vi "Arm Hardware.vi"(8 "error in (no error)":errorcluster, 9 "Request type":T1=enum."User command", 11 "Red Pitaya Digitizer in":refnum<class "Red Pitaya Digitizer.lvclass">) -> (0 "error out":errorcluster, 3 "Red Pitaya Digitizer out":refnum<class "Red Pitaya Digitizer.lvclass">)   [LabVIEW 2024, in "Red Pitaya Digitizer.lvclass"]
uses:
  Red Pitaya Digitizer.lvclass
  C:/GitHub/NHMFL_Core/Libraries/Instruments/Pulse Driver/Lockin Digitizer Driver/Lockin Digitizer Driver.lvclass
  C:/GitHub/NHMFL_Core/Libraries/Instruments/Pulse Driver/Pulse Driver.lvclass
  Red Pitaya Digitizer.lvclass/Red Pitaya Digitizer.ctl
  Instruments/Pulse Driver/Pulse Driver.lvclass/Pulse Driver.ctl
  RP Core/RP Instrument/RP Instrument.lvclass/RP Instrument.ctl
  RP Core/RP Instrument/RP Instrument.lvclass
  <vilib>/Utility/miscctls.llb/LVMapReplaceAction.ctl
  LabActor/Controllers/Process Controller/Request type.ctl
panel:
  out "key not found?":bool
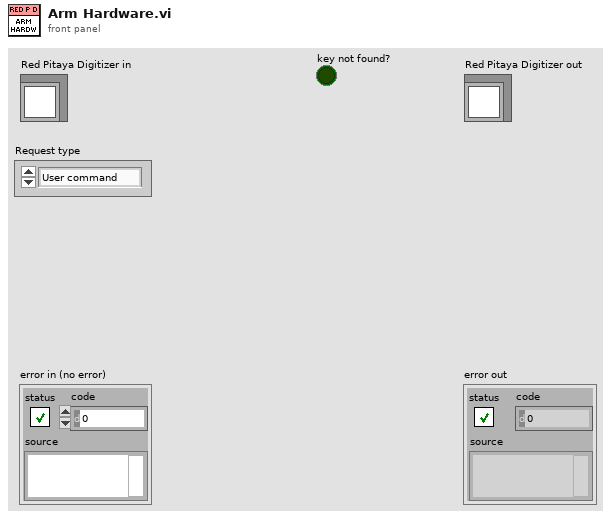
[diagram p1: front panel]
types:
  T1 = typedef "Request type.ctl" = enum16{"Process complete", "User command", "Auto-restart", "Error"}
  T2 = typedef "LVMapReplaceAction.ctl" = enum32{"Modify Entry only if found", "Add or Modify Entry", "Delete Entry"}
  T3 = typedef "Pusle Driver Configuration.ctl" = cluster{"Post-trigger delay":dbl, "Post-trigger duration":dbl, "Rate":dbl, "Ranges":dbl[], "Re-name channels":string[], "Active channels":string, "External clock":bool}
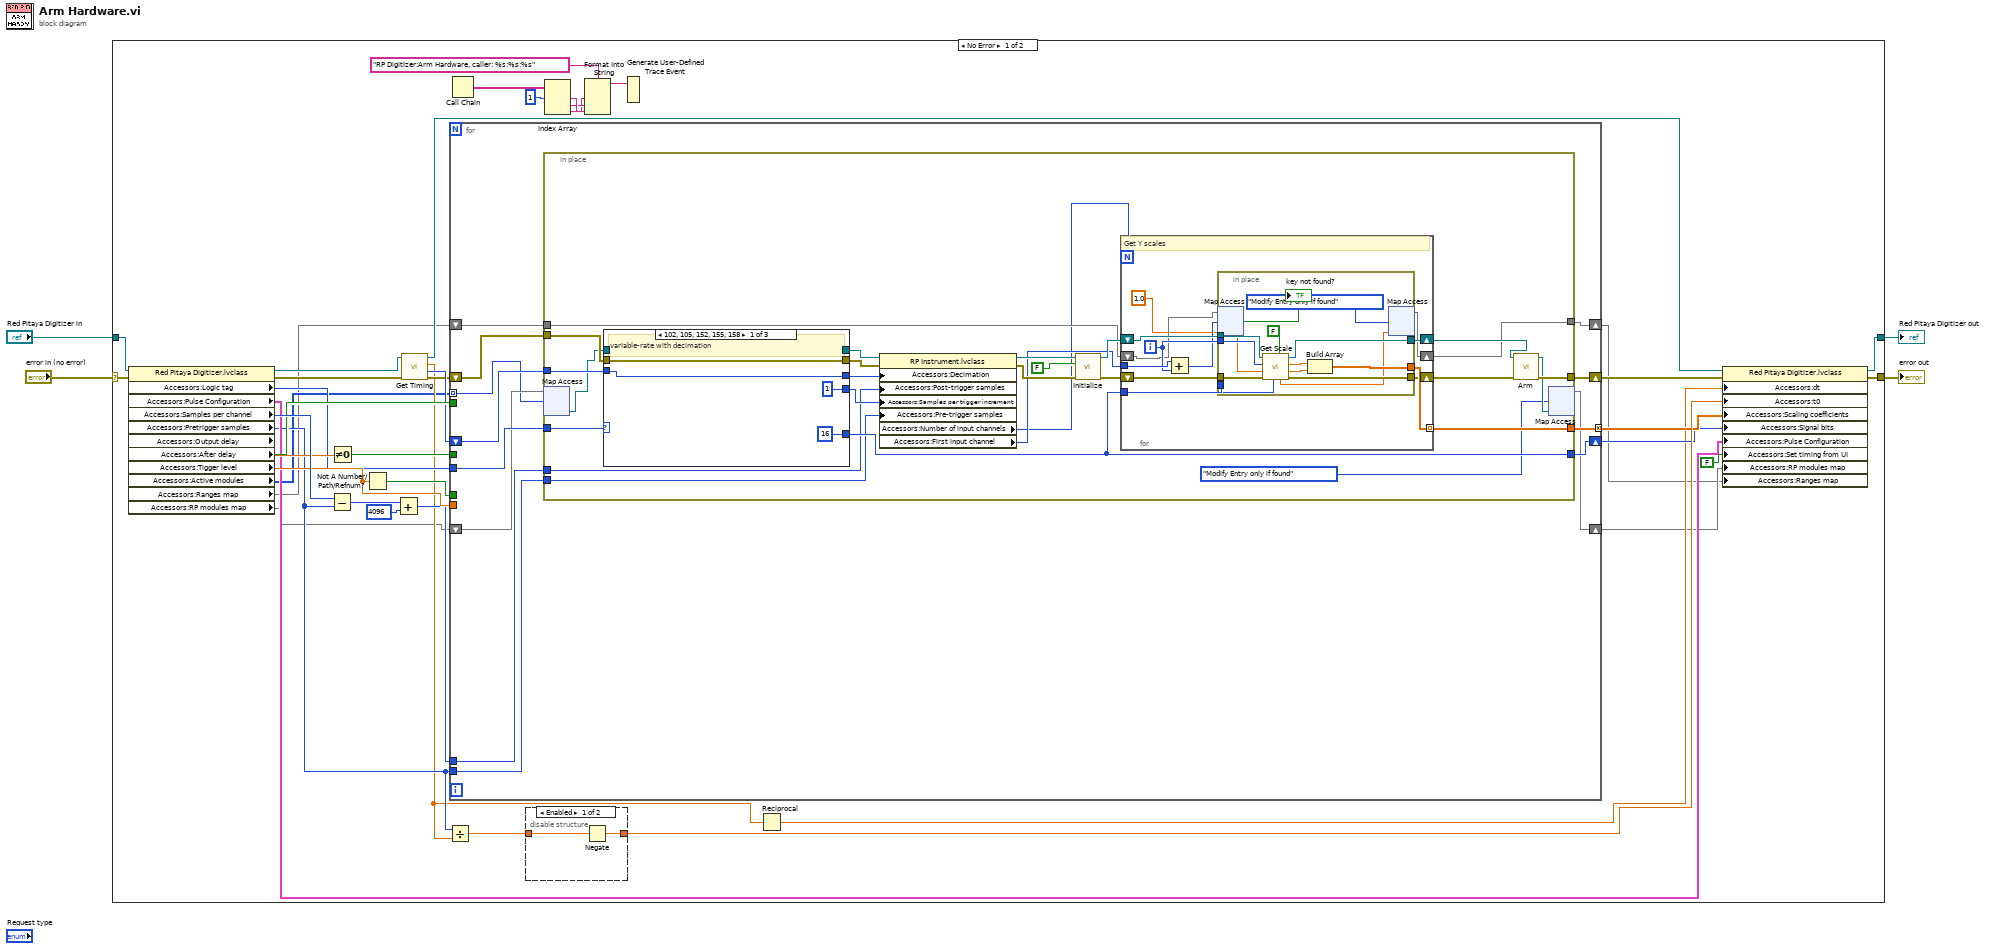
[diagram p0: block diagram]
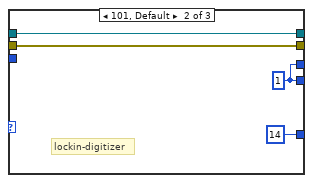
[diagram p3: hidden frame]
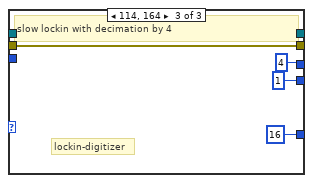
[diagram p4: hidden frame]
diagram:
  n1 = case shown="No Error" "error in (no error)" {
    selector: "error in (no error)" -> [w36 w128]
    tunnel: "Red Pitaya Digitizer in" -> [w45 w129]
    tunnel: [w41 w128] -> w2
    tunnel: [w40 w129] -> w1
    frame No Error {
      n2 = property class="Red Pitaya Digitizer.lvclass"(reference=w45, error in=w36) -> (reference out=w23:refnum<class "Red Pitaya Digitizer.lvclass">, error out=w26:errorcluster, "Accessors:Logic tag"=w28:u16, "Accessors:Pulse Configuration"=w21:T3, "Accessors:Samples per channel"=w44:i32, "Accessors:Pretrigger samples"=w11:i32, "Accessors:Output delay"=w33:dbl, "Accessors:After delay"=w32:bool, "Accessors:Tigger level"=w30:dbl, "Accessors:Active modules"=w9:i32[], "Accessors:Ranges map"=w8:map{i32, dbl}, "Accessors:RP modules map "=w7:map{i32, refnum<class "RP Instrument.lvclass">})
      n3 = Subtract(x=w44, y=w11) -> (x-y=w43:i32)
      n4 = Not Equal To 0?(x=w33) -> (x != 0?=w34:bool)
      n5 = Not A Number/Path/Refnum?(number/path/refnum=w30) -> (NaN/Path/Refnum?=w31:bool)
      n6 = Add(x=w43, y=4096) -> (x+y=w13:i32)
      n7 = call-dynamic "Get Timing.vi"("error in (no error)"=w26, "Red Pitaya Digitizer in"=w23) -> ("error out"=w24:errorcluster, "Decimation"=w25:i32, "Rate"=w10:dbl, "Red Pitaya Digitizer out"=w22:refnum<class "Red Pitaya Digitizer.lvclass">)  [unwired: 6 in]
      n8 = Divide(x=w11, y=w10) -> (x/y=w39:dbl)
      n9 = for {
        tunnel: w13 -> [w61]
        tunnel: [w59] -> w37 mode=concatenating
        tunnel: w28 -> [w57]
        tunnel: w34 -> [_]
        tunnel: w32 -> [_]
        tunnel: w31 -> [_]
        tunnel: w30 -> [_]
        shift-right: [w60] -> w42
        shift-left: w24 -> [w56]
        shift-right: [w58] -> w35
        shift-left: w25 -> [w55]
        tunnel: w11 -> [w54]
        tunnel: w9 -> [w51] mode=indexing
        shift-right: [w50] -> w6
        shift-left: w7 -> [w52]
        shift-right: [w49] -> w5
        shift-left: w8 -> [w53]
        n10 = in-place {
          in-place-border: w61 -> [w64]
          in-place-border: [w85] -> w60
          in-place-border: [w84] -> w59
          in-place-border: [w82] -> w58
          in-place-border: w57 -> [w81]
          in-place-border: w56 -> [w76]
          in-place-border: w55 -> [w73]
          in-place-border: w54 -> [w72]
          in-place-border: w53 -> [w70]
          in-place-border: [w62] -> w49
          n11 = in-place-map #1(w52, w51) -> (w67:refnum<class "RP Instrument.lvclass">)  [unwired: 1 in, 1 out]
          n12 = case shown="102, 105, 152, 155, 158" w81 {
            tunnel: [16 ("Signal bits") 14 ("Signal bits") 16 ("Signal bits")] -> w82
            tunnel: [1 ("Samples per trigger increment") w93 1 ("Samples per trigger increment")] -> w83
            tunnel: w73 -> [w88 _ _]
            tunnel: w67 -> [w90 w95 w99]
            tunnel: [w90 w95 w99] -> w75
            tunnel: w76 -> [w89 w94 w98]
            tunnel: [w89 w94 w98] -> w74
            tunnel: [w88 w93 4 ("Samples per trigger increment")] -> w63
            frame 102, 105, 152, 155, 158 {
              # "variable-rate with decimation"
            }
            frame 101, Default {
              w93 = 1 ("Samples per trigger increment")
              # "lockin-digitizer"
            }
            frame 114, 164 {
              # "lockin-digitizer"
              # "slow lockin with decimation by 4"
            }
          }
          n13 = property class="RP Instrument.lvclass"(reference=w75, error in=w74, "Accessors:Decimation"=w63, "Accessors:Post-trigger samples"=w64, "Accessors:Samples per trigger increment "=w83, "Accessors:Pre-trigger samples"=w72) -> (reference out=w87:refnum<class "RP Instrument.lvclass">, error out=w86:errorcluster, "Accessors:Number of input channels"=w68:i32, "Accessors:First input channel"=w69:i32)
          n14 = call-dynamic "Initialize.vi"("error in (no error)"=w86, "Reset"=FALSE, "RP Instrument in"=w87) -> ("error out"=w79:errorcluster, "RP Instrument out"=w80:refnum<class "RP Instrument.lvclass">)  [unwired: 7 in]
          n15 = for {
            N: w68 -> [_]
            tunnel: [w113] -> w84 mode=indexing
            tunnel: w82 -> [w110]
            shift-right: [w109] -> w77
            shift-left: w80 -> [w112]
            shift-right: [w108] -> w78
            shift-left: w79 -> [w111]
            tunnel: w69 -> [w107]
            shift-right: [w102] -> w62
            shift-left: w70 -> [w105]
            i -> [w106]
            # "Get Y scales"
            n16 = Add(x=w107, y=w106) -> (x+y=w104:i32)
            n17 = in-place {
              in-place-border: [w127] -> w113
              in-place-border: w112 -> [w126]
              in-place-border: w111 -> [w125]
              in-place-border: w110 -> [w122]
              in-place-border: [w121] -> w109
              in-place-border: [w120] -> w108
              in-place-border: w106 -> [w119]
              n18 = in-place-map #2(w105, w104, 1.0 ("default value")) -> (w117:dbl, →"key not found?":bool)
              n19 = call-dynamic "Get Scale.vi"("Read calibration"=FALSE, "Signal bits"=w122, "error in (no error)"=w125, "Range"=w117, "Channel"=w119, "RP Instrument in"=w126) -> ("error out"=w120:errorcluster, "slope"=w123:dbl, "y intersept"=w124:dbl, "RP Instrument out"=w121:refnum<class "RP Instrument.lvclass">, "Actual range"=w116:dbl)  [unwired: 1 in]
              n20 = Build Array(w124, w123) -> (w127:dbl[])
              n21 = in-place-map #2(w116, LVMapReplaceAction."Modify Entry only if found" ("action")) -> (w102:map{i32, dbl})  [unwired: 2 out]
            }
          }
          n22 = call-dynamic "Arm.vi"("error in (no error)"=w78, "RP Instrument in"=w77) -> ("error out"=w85:errorcluster, "RP Instrument out"=w66:refnum<class "RP Instrument.lvclass">)  [unwired: 8 in]
          n23 = in-place-map #1(w66, LVMapReplaceAction."Modify Entry only if found" ("action")) -> (w50:map{i32, refnum<class "RP Instrument.lvclass">})  [unwired: 2 out]
        }
      }
      n24 = Call Chain() -> (call chain=w19:string[])
      n25 = disable-structure shown="Enabled" {
        disable-tunnel: w39 -> [w47 w48]
        disable-tunnel: [w46 w48] -> w38
        frame Enabled {
          n26 = Negate(x=w47) -> (-x=w46:dbl)
        }
        frame Disabled {
        }
      }
      n27 = Index Array(array=w19, index #1=1 ("index")) -> (element #1=w18:string, element #2=w17:string, element #3=w16:string)  [unwired: 2 in]
      n28 = Format Into String(format string="RP Digitizer:Arm Hardware, caller: %s:%s:%s" ("string"), w16, w17, w18) -> (resulting string=w14:string)  [unwired: 2 in, 1 out]
      n29 = Generate User-Defined Trace Event(2:w14) -> ()  [unwired: 1 in]
      n30 = Reciprocal(x=w10) -> (1/x=w27:dbl)
      n31 = property class="Red Pitaya Digitizer.lvclass"(reference=w22, error in=w42, "Accessors:dt"=w27, "Accessors:t0"=w38, "Accessors:Scaling coefficients"=w37, "Accessors:Signal bits"=w35, "Accessors:Pulse Configuration"=w21, "Accessors:Set timing from UI"=FALSE ("Set timing from UI"), "Accessors:RP modules map "=w6, "Accessors:Ranges map"=w5) -> (reference out=w40:refnum<class "Red Pitaya Digitizer.lvclass">, error out=w41:errorcluster)
    }
    frame Error {
    }
  }
  "error out" <- w2
  "Red Pitaya Digitizer out" <- w1
